vi "Parse CSV (Polymorphic).vi"   [LabVIEW 2012]
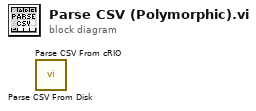
[diagram p0: block diagram]
diagram:
  n1 = call "Parse CSV From Disk.vi"() -> ()  [unwired: 5 in, 1 out]
  n2 = call "Parse CSV From cRIO.vi"() -> ()  [unwired: 5 in, 1 out]
